vi "Translate Element Names.vi"(11 "Element Name":string) -> (3 "Translated Element Name to Basic Name":string)   [LabVIEW 2014]
doc: "Translate element name. For developing there are used elements names, like \"WhileLoop\",\"Foloop\" but sometimes something is not running correctly so if there is use of some special name like \"TopConstant\" which is not name used by LabVIEW, using this VI will translate name \"TopConstant\" ---> \"Constant\" what is wanted behaviour."
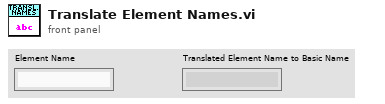
[diagram p1: front panel]
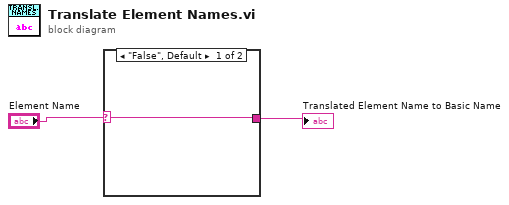
[diagram p0: block diagram]
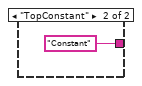
[diagram p2: hidden frame]
diagram:
  n1 = case shown="\"False\", Default" "Element Name" {
    selector: "Element Name" -> [w3 _]
    tunnel: [w3 "Constant"] -> w1
    frame "False", Default {
    }
    frame "TopConstant" {
    }
  }
  "Translated Element Name to Basic Name" <- w1
